vi "VI Tree.vi"() -> ()   [LabVIEW 2020, in "Active Technologies AWG3000.lvlib"]
doc: "This is the instrument driver for the <B>Tektronix AFG 300 Series</B>. The VI Tree displays all the user-callable VIs of the instrument driver in an organized table."
uses:
  Active Technologies AWG3000.lvlib
panel:
  in  "VISA resource name":refnum<visa-resource-name>
  # "SEE DIAGRAM\nFOR VI TREE."
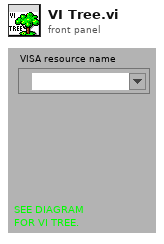
[diagram p1: front panel]
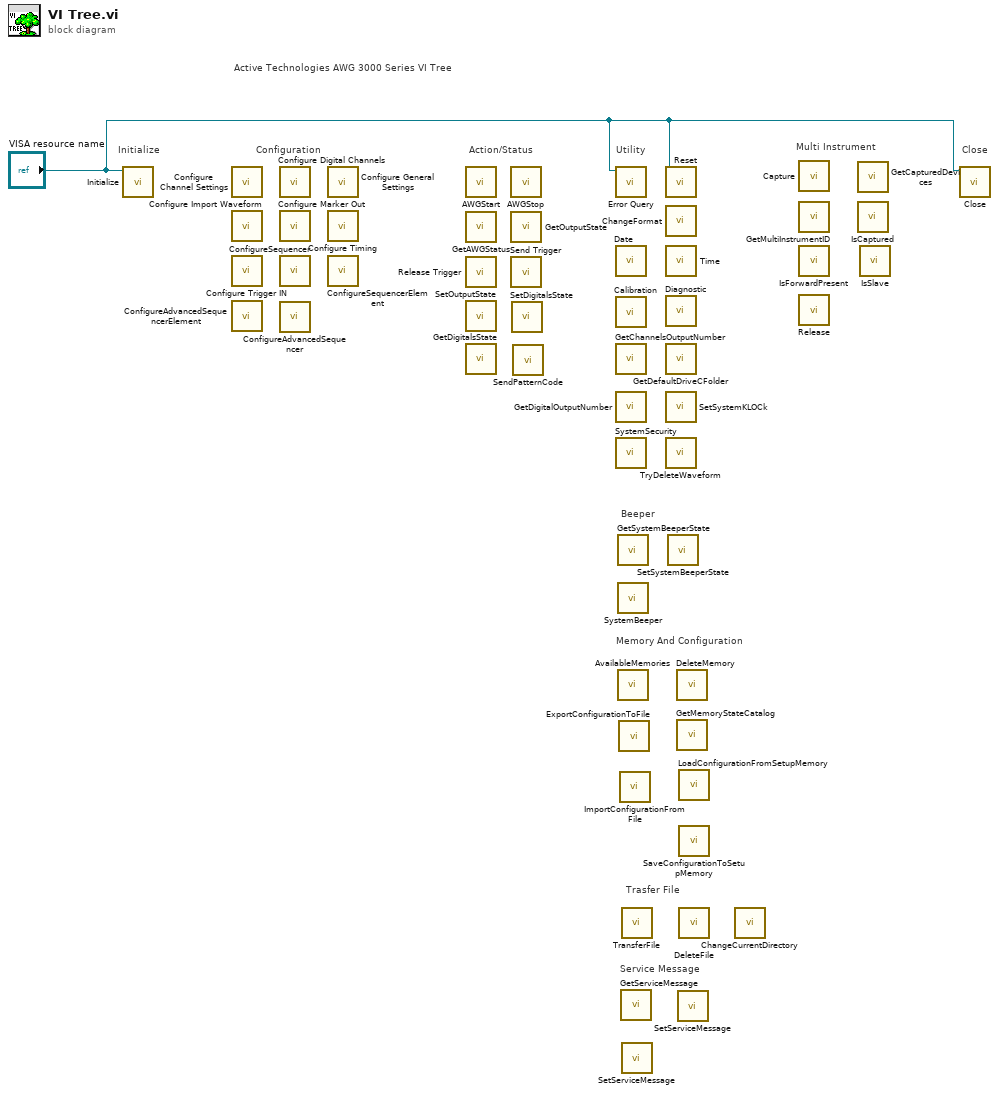
[diagram p0: block diagram]
diagram:
  # "Multi Instrument"
  # "Service Message"
  # "Trasfer File"
  # "Memory And Configuration"
  # "Beeper"
  # "Active Technologies AWG 3000 Series VI Tree"
  # "Configuration"
  # "Utility"
  # "Action/Status"
  # "Close"
  # "Initialize"
  n1 = call "Initialize.vi"("VISA resource name"="VISA resource name") -> ()  [unwired: 5 in, 6 out]
  n2 = call "Configure Channel Settings.vi"() -> ()  [unwired: 14 in, 2 out]
  n3 = call "Configure Import Waveform.vi"() -> ()  [unwired: 8 in, 2 out]
  n4 = call "Configure Trigger IN.vi"() -> ()  [unwired: 18 in, 2 out]
  n5 = call "ConfigureAdvancedSequencerElement.vi"() -> ()  [unwired: 6 in, 2 out]
  n6 = call "Configure Digital Channels.vi"() -> ()  [unwired: 8 in, 2 out]
  n7 = call "Configure Marker Out.vi"() -> ()  [unwired: 8 in, 2 out]
  n8 = call "ConfigureSequencer.vi"() -> ()  [unwired: 4 in, 2 out]
  n9 = call "ConfigureAdvancedSequencer.vi"() -> ()  [unwired: 4 in, 2 out]
  n10 = call "Configure General Settings.vi"() -> ()  [unwired: 9 in, 2 out]
  n11 = call "Configure Timing.vi"() -> ()  [unwired: 7 in, 2 out]
  n12 = call "ConfigureSequencerElement.vi"() -> ()  [unwired: 6 in, 2 out]
  n13 = call "AWGStart.vi"() -> ()  [unwired: 2 in, 2 out]
  n14 = call "GetAWGStatus.vi"() -> ()  [unwired: 2 in, 4 out]
  n15 = call "Release Trigger.vi"() -> ()  [unwired: 2 in, 2 out]
  n16 = call "SetOutputState.vi"() -> ()  [unwired: 4 in, 2 out]
  n17 = call "GetDigitalsState.vi"() -> ()  [unwired: 2 in, 3 out]
  n18 = call "AWGStop.vi"() -> ()  [unwired: 2 in, 2 out]
  n19 = call "GetOutputState.vi"() -> ()  [unwired: 3 in, 3 out]
  n20 = call "Send Trigger.vi"() -> ()  [unwired: 2 in, 2 out]
  n21 = call "SetDigitalsState.vi"() -> ()  [unwired: 3 in, 2 out]
  n22 = call "SendPatternCode.vi"() -> ()  [unwired: 3 in, 2 out]
  n23 = call "Error Query.vi"("VISA resource name"="VISA resource name") -> ()  [unwired: 7 in, 4 out]
  n24 = call "Date.vi"() -> ()  [unwired: 2 in, 3 out]
  n25 = call "Calibration.vi"() -> ()  [unwired: 2 in, 3 out]
  n26 = call "GetChannelsOutputNumber.vi"() -> ()  [unwired: 2 in, 3 out]
  n27 = call "GetDigitalOutputNumber.vi"() -> ()  [unwired: 2 in, 3 out]
  n28 = call "SystemSecurity.vi"() -> ()  [unwired: 2 in, 2 out]
  n29 = call "GetSystemBeeperState.vi"() -> ()  [unwired: 3 in, 2 out]
  n30 = call "SystemBeeper.vi"() -> ()  [unwired: 2 in, 2 out]
  n31 = call "AvailableMemories.vi"() -> ()  [unwired: 2 in, 3 out]
  n32 = call "ExportConfigurationToFile.vi"() -> ()  [unwired: 3 in, 2 out]
  n33 = call "ImportConfigurationFromFile.vi"() -> ()  [unwired: 3 in, 2 out]
  n34 = call "GetServiceMessage.vi"() -> ()  [unwired: 2 in, 3 out]
  n35 = call "TransferFile.vi"() -> ()  [unwired: 6 in, 2 out]
  n36 = call "SetServiceMessage.vi"() -> ()  [unwired: 3 in, 2 out]
  n37 = call "Reset.vi"("VISA resource name"="VISA resource name") -> ()  [unwired: 9 in, 2 out]
  n38 = call "ChangeFormat.vi"() -> ()  [unwired: 3 in, 2 out]
  n39 = call "Time.vi"() -> ()  [unwired: 2 in, 3 out]
  n40 = call "Diagnostic.vi"() -> ()  [unwired: 2 in, 3 out]
  n41 = call "GetDefaultDriveCFolder.vi"() -> ()  [unwired: 2 in, 3 out]
  n42 = call "SetSystemKLOCk.vi"() -> ()  [unwired: 3 in, 2 out]
  n43 = call "TryDeleteWaveform.vi"() -> ()  [unwired: 3 in, 3 out]
  n44 = call "SetSystemBeeperState.vi"() -> ()  [unwired: 3 in, 2 out]
  n45 = call "DeleteMemory.vi"() -> ()  [unwired: 4 in, 2 out]
  n46 = call "GetMemoryStateCatalog.vi"() -> ()  [unwired: 2 in, 3 out]
  n47 = call "SetServiceMessage.vi"() -> ()  [unwired: 3 in, 2 out]
  n48 = call "LoadConfigurationFromSetupMemory.vi"() -> ()  [unwired: 4 in, 2 out]
  n49 = call "SaveConfigurationToSetupMemory.vi"() -> ()  [unwired: 4 in, 2 out]
  n50 = call "DeleteFile.vi"() -> ()  [unwired: 3 in, 2 out]
  n51 = call "ChangeCurrentDirectory.vi"() -> ()  [unwired: 3 in, 2 out]
  n52 = call "Capture.vi"() -> ()  [unwired: 2 in, 2 out]
  n53 = call "GetMultiInstrumentID.vi"() -> ()  [unwired: 3 in, 3 out]
  n54 = call "IsForwardPresent.vi"() -> ()  [unwired: 3 in, 3 out]
  n55 = call "Release.vi"() -> ()  [unwired: 2 in, 2 out]
  n56 = call "GetCapturedDevices.vi"() -> ()  [unwired: 3 in, 3 out]
  n57 = call "IsCaptured.vi"() -> ()  [unwired: 3 in, 3 out]
  n58 = call "IsSlave.vi"() -> ()  [unwired: 3 in, 3 out]
  n59 = call "Close.vi"("VISA resource name"="VISA resource name") -> ()  [unwired: 10 in, 1 out]
